vi "DjtgGetSpeed.vi"(8 "Error In":errorcluster, 11 "Device Number":u32) -> (0 "Error Out":errorcluster, 2 "JTAG Speed (Hz)":u32, 3 "Device Number":u32)   [LabVIEW 2011, in "LVH-Adept.lvlib" / "DJTG.lvlib"]
doc: "This function is used to get the current speed of the DJTG port. The value returned in pfrqCur is in\nHZ."
uses:
  <vilib>/LabVIEW Hacker/Adept/Private/DJTG/DJTG.lvlib
  <vilib>/LabVIEW Hacker/Adept/Private/DJTG/Private/Type Defs/Error.ctl
  <vilib>/LabVIEW Hacker/Adept/Private/Resources/djtg.dll
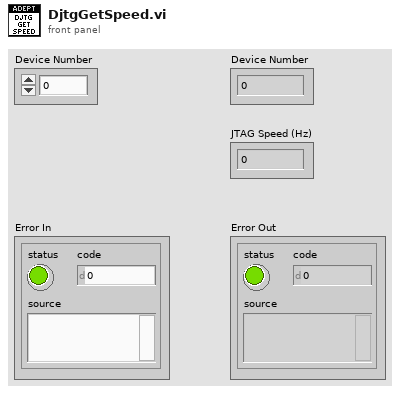
[diagram p1: front panel]
types:
  T1 = typedef "LVH-Adept.lvlib/DJTG.lvlib/Error.ctl" = enum16{"Unknown", "Enable", "PutTmsTdiBits", "GetTdoBits", "Disable", "Close", "Set Aux Reset", "Port Properties", "Get Speed", "Set Speed", "Get Port Count", "Get Batch Properties", "Enable Port", "Set Tmd Tdi Tck", "Get Tms Tdi Tdo Tck", "Put Tdi Bits", "Put Tms Bits", "Clock Tck", "Wait", "Batch", "Flash FPGA"}
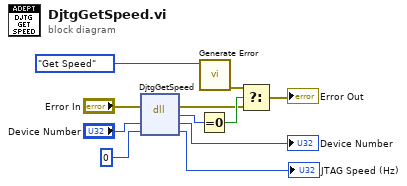
[diagram p0: block diagram]
diagram:
  n1 = dll-call lib="C:/Program Files (x86)/National Instruments/LabVIEW 2011/vi.lib/LabVIEW Hacker/Adept/Private/Resources/djtg.dll" fn="DjtgGetSpeed"(error in="Error In", "hif"="Device Number", "pfrqCur"=u32 0) -> (error out=w6:errorcluster, "Success"=w5:u32, "hif"=→"Device Number":u32, "pfrqCur"=→"JTAG Speed (Hz)":u32)  [unwired: 2 in, 1 out]
  n2 = Equal To 0?(x=w5) -> (x = 0?=w11:bool)
  n3 = call <vilib>:"Generate Error.vi"("DJTG Error"=Error."Get Speed") -> ("Error Out"=w10:errorcluster)  [unwired: 10 in]
  n4 = Select(t=w10, s=w11, f=w6) -> (s? t:f=→"Error Out":errorcluster)
